vi "ATS_Async_Buffer_Size.vi"(8 "ReadSamples":T3, 9 "Async_Setting":T1, 10 "Channel":T2, 11 "DeviceIn":i32) -> (0 "ReadSamples_Out":T3, 1 "RecordsPerBuffer_Out":u32, 2 "Handle":u32, 3 "DeviceOut":i32, 4 "BufferSize":u32, 5 "#Bytes/Sample":u32)   [LabVIEW 2010]
doc: "_____AlazarTech, Scope_____\n\nEvaluate the Buffer size require for the AsyncDMA transfer mode.\nThe uBytesToRead parameter must be equal to the size of the AutoDMA transfer in bytes, which can be calculated as follows:\n· If the ADMA_ENABLE_HEADERS flag was set, then the size the record header in samples is: \n record_header_size_samples = 16 bytes / bytes_per_sample;\nIf the ADMA_ENABLE_HEADERS flag was not set, then the size of the record the size of the record header in samples is zero. \n record_header_size_samples = 0;\n· The number of bytes per record is given by: \n bytes_per_record = bytes_per_sample * (record_header_size_samples +\n samples_per_record);\n· The number of bytes per transfer is given by:\n bytes_per_transfer = number_of_enabled_channels *\n bytes_per_record * records_per_transfer;"
uses:
  ATS_ctl/ATS_ReadSamples.ctl
  ATS_ctl/ATS_DMA_Channel.ctl
  ATS_ctl/ATS_Async_Setting.ctl
  ATS_ctl/ATS_Global_Ctrl.ctl
panel:
  # "If Length = 0 ==> Memory size."
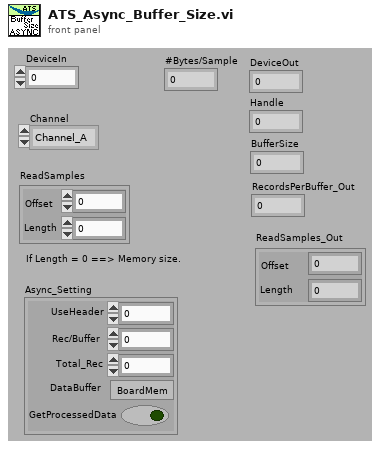
[diagram p1: front panel]
types:
  T1 = typedef "ATS_Async_Setting.ctl" = cluster{"UseHeader":u32, "Rec/Buffer":u32, "Total_Rec":u32, "DataBuffer":bool, "GetProcessedData":bool}
  T2 = typedef "ATS_DMA_Channel.ctl" = enum16{"Channel_A", "Channel_B", "A & B"}
  T3 = typedef "ATS_ReadSamples.ctl" = cluster{"Offset":i32, "Length":u32}
  T4 = typedef "ATS_Global_Ctrl.ctl" = enum16{"Init_Device", "Clear_ALL", "Set", "Get"}
  T5 = typedef "ATS_Global_4Ch.ctl" = cluster{"Record":T6, "Clock":T7, "Inputs":T11, "Trigger":T17}
  T6 = typedef "Record.ctl" = cluster{"Count":u32, "Presize":u32, "Length":u32}
  T7 = typedef "Clock.ctl" = cluster{"ClckSource":T8, "ClckRate":T9, "ClckEdge":T10, "Decimation":u32}
  T8 = typedef "ClockSource.ctl" = enum16{"Internal", "External", "Medium Ext.", "Slow Ext.", "Ext. AC", "Ext. DC", "Ext. (PLL)"}
  T9 = typedef "ClockRate.ctl" = u32
  T10 = typedef "ClockEdge.ctl" = u16
  T11 = typedef "ATS_InputArray.ctl" = T12[]
  T12 = typedef "InputCtrl.ctl" = cluster{"Coupling":T13, "Range":T14, "Impedance":T15, "Bandwidth":T16}
  T13 = typedef "Coupling.ctl" = enum16{"AC", "DC"}
  T14 = typedef "Range.ctl" = u32
  T15 = typedef "Impedance.ctl" = enum16{"1M ohms", "50 ohms"}
  T16 = typedef "Bandwidth.ctl" = enum16{"Full Bandwidth", "Reduce Bandwidth"}
  T17 = typedef "ATS_Trigger_4Ch.ctl" = cluster{"TrigOperation":T18, "Timeout (s)":dbl, "Trig. Delay":u32, "Engine X":T19, "Engine Y":T19, "ExtTrigControl":T21}
  T18 = typedef "TriggerOperation.ctl" = enum16{"Only X", "Only Y", "X or Y", "X and Y", "X xor Y", "X and not Y", "not X and Y"}
  T19 = typedef "ATS_TriggerEngine_4Ch.ctl" = cluster{"Source":T20, "Slope":enum32{"Positive", "Negative"}, "Level":u32}
  T20 = typedef "ATS_TriggerSource_4Ch.ctl" = enum32{"Chan_A", "Chan_B", "External", "Disable", "Chan_C", "Chan_D"}
  T21 = typedef "ExtTrigger.ctl" = cluster{"Coupling":T13, "Range":T22}
  T22 = typedef "ExtTrigRange.ctl" = enum16{"1 V", "5 V", "TTL"}
  T23 = typedef "Device_Info.ctl" = cluster{"Handle":u32, "Board":string, "CPLD":string, "MemorySize":u32, "SampleSize":u8, "ID":i32, "High_Memory":bool, "Chan/Board":u8}
  T24 = typedef "ATS_Global_Specs_Ctrl.ctl" = cluster{"ClckSource":cluster{"Internal":bool, "External":bool, "Medium Ext.":bool, "Slow Ext.":bool, "Ext. AC":bool, "Ext. DC":bool, "Ext. (PLL)":bool}, "ClckRate":cluster{"1 kS/s":bool, "2 kS/s":bool, "5 kS/s":bool, "10 kS/s":bool, "20 kS/s":bool, "50 kS/s":bool, "100 kS/s":bool, "200 kS/s":bool, "500 kS/s":bool, "1 MS/s":bool, "2 MS/s":bool, "5 MS/s":bool, "10 MS/s":bool, "20 MS/s":bool, "25 MS/s":bool, "50 MS/s":bool, "100 MS/s":bool, "125 MS/s":bool, "160 MS/s":bool, "180 MS/s":bool, "200 MS/s":bool, "250 MS/s":bool, "500 MS/s":bool, "1 GS/s":bool}, "ClckEdge":cluster{"Rising":bool, "Falling":bool}, "InputCoupling":cluster{"AC":bool, "DC":bool}, "InputRange":cluster{"20mV":bool, "40mV":bool, "50mV":bool, "80mV":bool, "100mV":bool, "200mV":bool, "400mV":bool, "500mV":bool, "800mV":bool, "1 V":bool, "2 V":bool, "4 V":bool, "5 V":bool, "8 V":bool, "10 V":bool, "16 V":bool, "20 V":bool, "40 V":bool, "HiFi":bool, "1.25 V":bool}, "Impedance":cluster{"1M ohms":bool, "50 ohms":bool, "300 ohms":bool}, "Bandwidth":cluster{"Full":bool, "Reduce":bool}, "RangeLim(50)":string, "AsyncDMA":cluster{"OnBoard":bool, "FPGA":bool}, "Memory":cluster{"VerifMem":bool, "HighMem":bool, "Combine":bool, "HighRecord":bool}, "ExtTrigCoupling":cluster{"AC":bool, "DC":bool}, "ExtTrigRange":cluster{"1 V":bool, "5 V":bool, "\nTTL":bool}, "AUX_IO_Trig":cluster{"Trig_Out":bool, "Trig_In":bool}, "AUX_IO_Slope":cluster{"Rising":bool, "Falling":bool}, "MaxPretrig":cluster{"MEM":u32, "FIFO":u32}, "AUX_I/O_Trig":cluster{"OUT_Trigger":bool, "OUT_PACER":bool, "OUT_BUSY":bool, "OUT_CLOCK":bool, "OUT_RESERVED":bool, "OUT_CAPTURE_ALMOST_DONE":bool, "OUT_AUXILIARY":bool, "OUT_SERIAL_DATA":bool, "IN_TRIGGER_ENABLE":bool, "IN_DIGITAL_TRIGGER":bool, "IN_GATE":bool, "IN_CAPTURE_ON_DEMAND":bool, "IN_RESET_TIMESTAMP":bool, "IN_SLOW_EXTERNAL_CLOCK":bool, "INPUT_AUXILIARY":bool, "INPUT_SERIAL_DATA":bool}, "ChannelsPerBoard":u8}
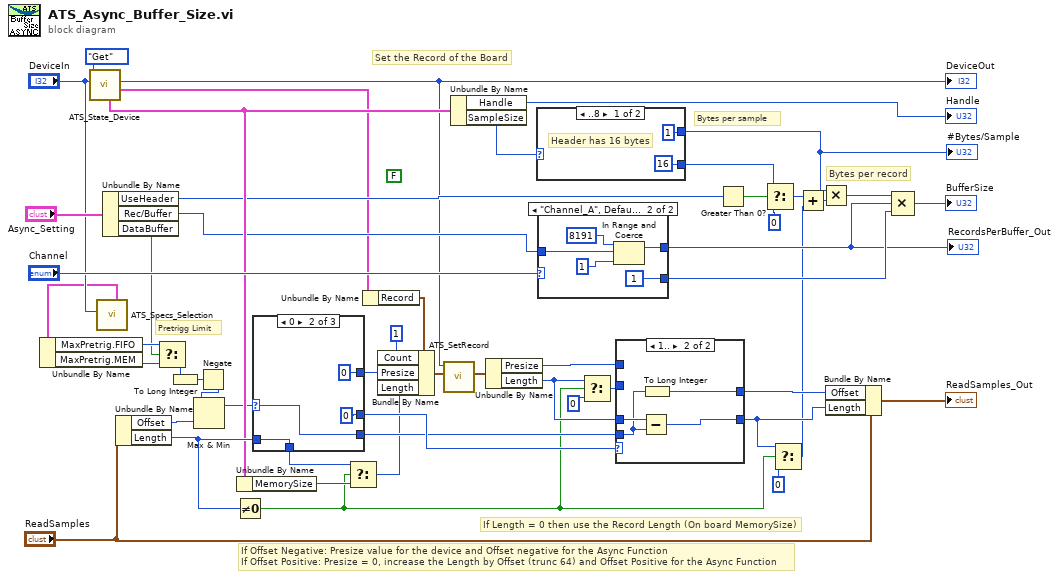
[diagram p0: block diagram]
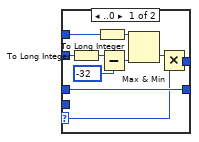
[diagram p2: hidden frame]
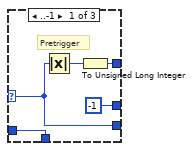
[diagram p3: hidden frame]
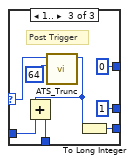
[diagram p4: hidden frame]
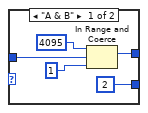
[diagram p5: hidden frame]
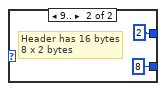
[diagram p6: hidden frame]
diagram:
  (unwired) FALSE ("Set_Manually (F)")
  # "Pretrigg Limit"
  # "If Offset Negative: Presize value for the device and Offset negative for the Async Function\nIf Offset Positive: Presize = 0, increase the Length by Offset (trunc 64) and Offset Positive for the Async Function"
  # "Set the Record of the Board"
  # "Bytes per record"
  # "Bytes per sample"
  # "If Length = 0 then use the Record Length (On board MemorySize)"
  n1 = call "ATS_State_Device.vi"("DeviceIn"="DeviceIn", "ATS_GBL_Ctrl"=ATS_Global_Ctrl."Get") -> ("SetupOut"=w3:T5, "DeviceOut"=w1:i32, "DevInfo_Out"=w19:T23)  [unwired: 4 in, 3 out]
  "DeviceOut" <- w1
  n2 = call "ATS_Specs_Selection.vi"("Device"="DeviceIn") -> ("Specifications"=w14:T24)  [unwired: 4 in, 6 out]
  n3 = Unbundle By Name(w14) -> ("MaxPretrig.FIFO"=w12:u32, "MaxPretrig.MEM"=w11:u32)
  n4 = Unbundle By Name("Async_Setting") -> ("UseHeader"=w7:u32, "Rec/Buffer"=w6:u32, "DataBuffer"=w8:bool)
  n5 = Unbundle By Name("ReadSamples") -> ("Offset"=w16:i32, "Length"=w30:u32)
  n6 = Select(t=w12, s=w8, f=w11) -> (s? t:f=w13:u32)
  n7 = To Long Integer(number=w13) -> (32bit integer=w9:i32)
  n8 = Negate(x=w9) -> (-x=w10:i32)
  n9 = Max & Min(x=w10, y=w16) -> (max(x,y)=w17:i32)  [unwired: 1 out]
  n10 = Not Equal To 0?(x=w30) -> (x != 0?=w21:bool)
  n11 = Unbundle By Name(w19) -> ("MemorySize"=w29:u32)
  n12 = case shown="0" w17 {
    selector: w17 -> [w53 w58 w64]
    tunnel: w30 -> [w56 w59 w69]
    tunnel: [w54 u32 0 ("Offset") u32 0 ("Offset")] -> w32
    tunnel: [w56 w59 w67] -> w27
    tunnel: [-1 ("-1, 0, 1") 0 ("-1, 0, 1") 1 ("-1, 0, 1")] -> w33
    tunnel: [w53 w58 w62] -> w31
    frame ..-1 {
      # "Pretrigger"
      n13 = Absolute Value(x=w53) -> (abs(x)=w57:i32)
      n14 = To Unsigned Long Integer(number=w57) -> (unsigned 32bit integer=w54:u32)
    }
    frame 0 {
    }
    frame 1.. {
      # "Post Trigger"
      n15 = call "ATS_Trunc.vi"("TruncValue"=u32 64, "Value"=w64) -> ("NewValue"=w63:u32)  [unwired: 5 in]
      n16 = Add(x=w63, y=w69) -> (x+y=w67:u32)
      n17 = To Long Integer(number=w63) -> (32bit integer=w62:i32)
    }
  }
  n18 = Select(t=w27, s=w21, f=w29) -> (s? t:f=w28:u32)
  n19 = Unbundle By Name(w3) -> ("Record"=w2:T6)
  n20 = Bundle By Name(cluster=w2, "Count"=u32 1 ("Record.Count"), "Presize"=w32, "Length"=w28) -> (w4:T6)
  n21 = call "ATS_SetRecord.vi"("RecordIn"=w4, "DeviceIn"=w1) -> ("RecordOut"=w5:T6)  [unwired: 7 in, 2 out]
  n22 = Unbundle By Name(w19) -> ("Handle"=→"Handle":u32, "SampleSize"=w50:u8)
  n23 = Unbundle By Name(w5) -> ("Presize"=w36:u32, "Length"=w26:u32)
  n24 = case shown="..8" w50 {
    tunnel: [u32 16 u32 8] -> w45
    tunnel: [u32 1 u32 2] -> w42
    frame ..8 {
      # "Header has 16 bytes"
    }
    frame 9.. {
      # "Header has 16 bytes\n8 x 2 bytes"
    }
  }
  "#Bytes/Sample" <- w42
  n25 = case shown="\"Channel_A\", Default" "Channel" {
    tunnel: [u32 2 ("Operation") u32 1 ("Operation")] -> w40
    tunnel: [w77 w80] -> w37
    tunnel: w6 -> [w75 w79]
    frame "A & B" {
      n26 = In Range and Coerce(upper limit=u32 4095, x=w75, lower limit=u32 1 ("x")) -> (coerced(x)=w77:u32)  [unwired: 1 out]
    }
    frame "Channel_A", Default {
      n27 = In Range and Coerce(upper limit=u32 8191, x=w79, lower limit=u32 1 ("x")) -> (coerced(x)=w80:u32)  [unwired: 1 out]
    }
  }
  "RecordsPerBuffer_Out" <- w37
  n28 = Select(t=w26, s=w21, f=u32 0) -> (s? t:f=w25:u32)
  n29 = case shown="1.." w33 {
    selector: w33 -> [w84 _]
    tunnel: w25 -> [w93 _]
    tunnel: w36 -> [w89 _]
    tunnel: [w86 w94] -> w35
    tunnel: w26 -> [w85 w97]
    tunnel: [w85 w96] -> w22
    tunnel: w31 -> [_ w95]
    frame ..0 {
      n30 = To Long Integer(number=w93) -> (32bit integer=w92:i32)
      n31 = To Long Integer(number=w89) -> (32bit integer=w88:i32)
      n32 = Subtract(x=w92, y=-32 ("value")) -> (x-y=w90:i32)
      n33 = Max & Min(x=w88, y=w90) -> (min(x,y)=w87:i32)  [unwired: 1 out]
      n34 = Multiply(x=w87, y=w84) -> (x*y=w86:i32)
    }
    frame 1.. {
      n35 = Subtract(x=w97, y=w95) -> (x-y=w96:u32)
      n36 = To Long Integer(number=w95) -> (32bit integer=w94:i32)
    }
  }
  n37 = Greater Than 0?(x=w7) -> (x > 0?=w48:bool)
  n38 = Select(t=w45, s=w48, f=u32 0 ("y")) -> (s? t:f=w44:u32)
  n39 = Select(t=w22, s=w21, f=u32 0) -> (s? t:f=w20:u32)
  n40 = Add(x=w44, y=w20) -> (x+y=w43:u32)
  n41 = Multiply(x=w42, y=w43) -> (x*y=w41:u32)
  n42 = Bundle By Name(cluster="ReadSamples", "Offset"=w35, "Length"=w22) -> (→"ReadSamples_Out":T3)
  n43 = Compound Arithmetic op=MULTIPLY(w41, w37, w40) -> (→"BufferSize":u32)
